vi "subsystem_ackCommand.vi"(8 "error in (no error)":errorcluster, 9 "ackcmd_Ctl":T1={"cmdSeqNum"=0, "ack"=0, "error"=0, "result"="                                                                                                                                                                                                                                                                "}, 10 "topic":string="Start", 11 "ProgrammaticInitialization in":refnum<class "ProgrammaticInitialization.lvclass">) -> (0 "error out":errorcluster, 3 "ProgrammaticInitialization out":refnum<class "ProgrammaticInitialization.lvclass">)   [LabVIEW 2016, in "ProgrammaticInitialization.lvclass"]
uses:
  ProgrammaticInitialization.lvclass
  ts_sallv_sedspectrometer/DataTypes/ackcmd.ctl
  commandType.ctl
  ProgrammaticInitialization.lvclass/ProgrammaticInitialization.ctl
  ts_sallv_sedspectrometer/SALLV_calibrationSpectrometer.lvlib
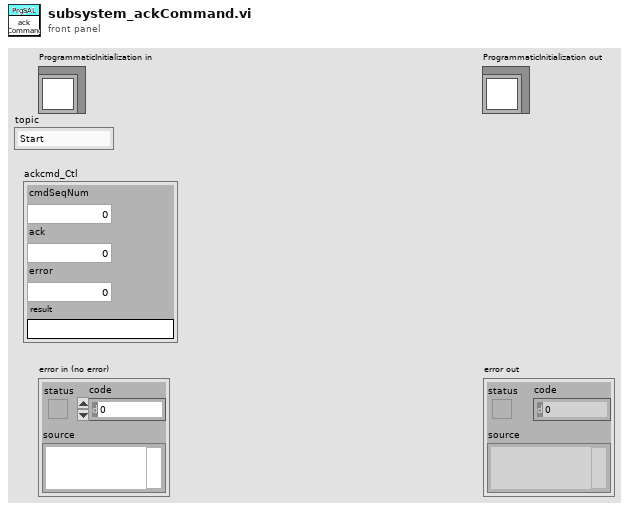
[diagram p1: front panel]
types:
  T1 = typedef "SALLV_calibrationSpectrometer.lvlib/ackcmd.ctl" = cluster{"cmdSeqNum":i32, "ack":i32, "error":i32, "result":string}
  T2 = typedef "ProgrammaticInitialization.lvclass/commandType.ctl" = enum16{"acceptCommand", "ackCommand", "cancelCallback_command", "cancelCallback_logEvent", "cancelCallback", "flushSamplesEvent", "getEvent", "getNextSample", "getResponse", "getSample", "issueCommand", "logEvent", "monitorCommand", "putSample", "registerCallback_command", "registerCallback_logEvent", "registerCallback", "salCommander", "salEvent", "salProcessor", "salTelemetrySub", "waitForCompletion"}
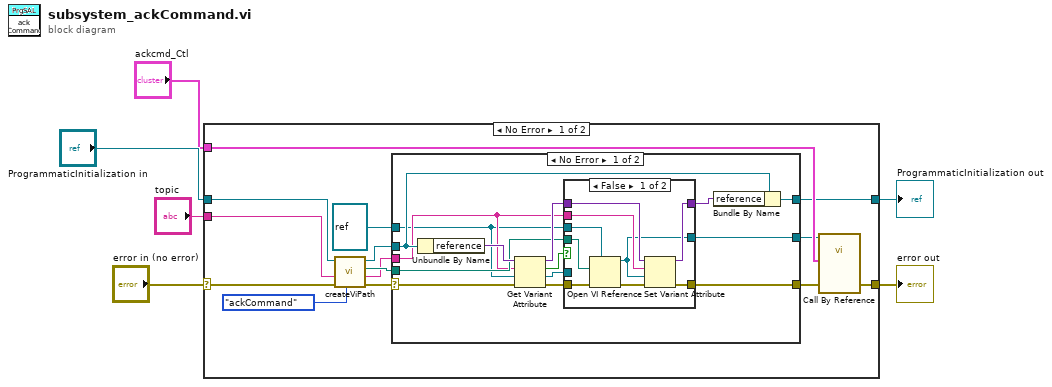
[diagram p0: block diagram]
diagram:
  n1 = case shown="No Error" "error in (no error)" {
    selector: "error in (no error)" -> [w19 w51]
    tunnel: [w16 w51] -> w5
    tunnel: [w7 w50] -> w3
    tunnel: "ProgrammaticInitialization in" -> [w8 w50]
    tunnel: "topic" -> [w18 _]
    tunnel: "ackcmd_Ctl" -> [w17 _]
    frame No Error {
      n2 = call "createViPath.vi"("CommandType"=commandType."ackCommand", "error in (no error)"=w19, "topic"=w18, "ProgrammaticInitialization in"=w8) -> ("error out"=w13:errorcluster, "vi name"=w11:string, "path"=w12:path, "ProgrammaticInitialization out"=w14:refnum<class "ProgrammaticInitialization.lvclass">)  [unwired: 4 in]
      n3 = case shown="No Error" w13 {
        selector: w13 -> [w31 w49]
        tunnel: [w30 w49] -> w10
        tunnel: [w26 w48] -> w7
        tunnel: w14 -> [w25 w48]
        tunnel: w11 -> [w23 _]
        tunnel: refnum<vi> refnum ("type specifier VI Refnum (for type only)") -> [w21 w47]
        tunnel: w12 -> [w24 _]
        tunnel: [w22 w47] -> w9
        frame No Error {
          n4 = Unbundle By Name(w25) -> ("reference"=w29:variant)
          n5 = Get Variant Attribute(Variant=w29, name=w23, default value (empty Variant)=w21, error in=w31) -> (duplicate Variant=w28:variant, found=w34:bool, value=w32:refnum<vi>, error out=w33:errorcluster)
          n6 = case shown="False" w34 {
            tunnel: w33 -> [w41 w46]
            tunnel: w32 -> [_ w44]
            tunnel: [w43 w46] -> w30
            tunnel: w28 -> [w36 w45]
            tunnel: [w42 w45] -> w27
            tunnel: w21 -> [w39 _]
            tunnel: w24 -> [w38 _]
            tunnel: w23 -> [w37 _]
            tunnel: [w35 w44] -> w22
            frame False {
              n7 = Open VI Reference(type specifier VI Refnum (for type only)=w39, vi path=w38, error in (no error)=w41) -> (vi reference=w35:refnum<vi>, error out=w40:errorcluster)  [unwired: 3 in]
              n8 = Set Variant Attribute(Variant=w36, name=w37, value=w35, error in=w40) -> (Variant out=w42:variant, error out=w43:errorcluster)  [unwired: 1 out]
            }
            frame True {
            }
          }
          n9 = Bundle By Name(cluster=w25, "reference"=w27) -> (w26:refnum<class "ProgrammaticInitialization.lvclass">)
        }
        frame Error {
        }
      }
      n10 = call-by-ref "?"(reference=w9, "error in (no error)"=w10, "ackcmd_Ctl"=w17) -> ("error out"=w16:errorcluster)  [unwired: 8 in, 4 out]
    }
    frame Error {
    }
  }
  "error out" <- w5
  "ProgrammaticInitialization out" <- w3
